vi "Producer-Consumer Example Test.vi"() -> ()   [LabVIEW 2019]
doc: "Use this template to build a producer/consumer design pattern with events to produce queue items. Use this design pattern instead of the user interface event handler pattern for user interfaces when you want to execute code asynchronously in response to an event without slowing the user interface responsiveness."
panel:
  out "LED":bool
  in  "Slide":dbl(slide) scale=0.0..10.0
  in  "Queue Event":bool
  in  "stop":bool
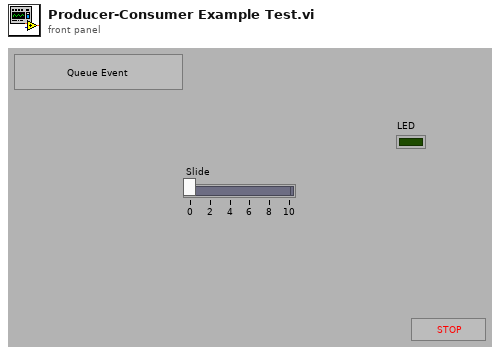
[diagram p1: front panel]
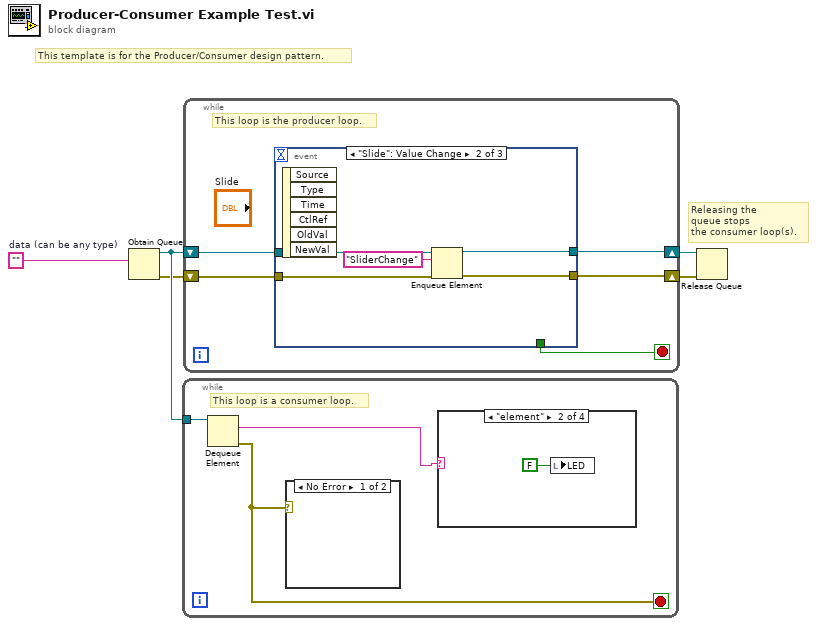
[diagram p0: block diagram]
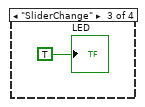
[diagram p3: hidden frame]
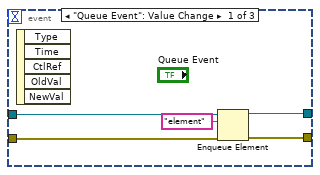
[diagram p6: hidden frame]
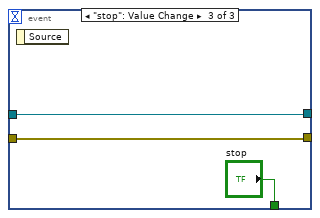
[diagram p7: hidden frame]
diagram:
  w1 = ""  # data (can be any type)
  # "Releasing the\nqueue stops\nthe consumer loop(s)."
  # "This template is for the Producer/Consumer design pattern."
  n1 = Obtain Queue(element data type=w1) -> (queue out=w5:refnum<queue>, error out=w4:errorcluster)  [unwired: 4 in, 1 out]
  n2 = while {
    tunnel: w5 -> [w8]
    stop <- w7 stop-if-true
    # "This loop is a consumer loop."
    n3 = Dequeue Element(queue=w8) -> (element=w6:string, error out=w7:errorcluster)  [unwired: 2 in, 2 out]
    n4 = case shown="No Error" w7 {
      frame No Error {
      }
      frame Error {
      }
    }
    n5 = case shown="\"element\"" w6 {
      frame "False", Default {
      }
      frame "element" {
        n6 = local write "LED"(FALSE ("LED")) -> ()
      }
      frame "SliderChange" {
        "LED" <- TRUE ("LED")
      }
      frame "True" {
      }
    }
  }
  n7 = while {
    shift-right: [w12] -> w2
    shift-left: w4 -> [w13]
    shift-right: [w14] -> w3
    shift-left: w5 -> [w15]
    stop <- w11 stop-if-true
    # "This loop is the producer loop."
    n8 = event shown="[1] \"Slide\": Value Change" {
      selector: _ -> [_ _ _]
      dyn-events: _ -> [_ _ _]
      timeout: _ -> [_ _ _]
      tunnel: w15 -> [w20 w24 w27]
      tunnel: [w19 w23 w27] -> w14
      tunnel: w13 -> [w18 w25 w26]
      tunnel: [w17 w22 w26] -> w12
      tunnel: [_ _ "stop"] -> w11
      event "Queue Event": Value Change {
        n9 = event-data() -> ()  [unwired: 1 in, 5 out]
        n10 = Enqueue Element(queue=w20, element="element", error in (no error)=w18) -> (queue out=w19:refnum<queue>, error out=w17:errorcluster)  [unwired: 1 in, 1 out]
      }
      event "Slide": Value Change {
        n11 = event-data() -> ()  [unwired: 1 in, 6 out]
        n12 = Enqueue Element(queue=w24, element="SliderChange", error in (no error)=w25) -> (queue out=w23:refnum<queue>, error out=w22:errorcluster)  [unwired: 1 in, 1 out]
      }
      event "stop": Value Change {
        n13 = event-data() -> ()  [unwired: 1 in, 1 out]
      }
    }
  }
  n14 = Release Queue(queue=w3, error in (no error)=w2) -> ()  [unwired: 1 in, 3 out]
